vi "Configure Capture Analyzer Measurement Write To File.vi"(8 "error in (no error)":errorcluster, 9 "Write to File (Off)":bool, 10 "Instance (1)":i32=1, 11 "VISA resource name":refnum<visa-resource-name>) -> (0 "error out":errorcluster, 3 "VISA resource name out":refnum<visa-resource-name>)   [LabVIEW 2015, in "Rohde&Schwarz CMXP GPRF.lvlib"]
doc: "Enables or disables saving of all buffer contents to files (I/Q data for all segments).\nWith <WriteToFolder> = ON, the files are stored when the capture buffer analyzer is started.\n\nAttribute:\nRSCMXPGPRF_ATTR_CAPTURE_ANALYZER_MEASUREMENT_WRITE_TO_FILE\n\nRemote-control command:\nCONFigure:GPRF:MEAS<i>:CANalyzer:SALL:WTFolder"
uses:
  <instrlib>/Rohde&Schwarz CMXP GPRF/Rohde&Schwarz CMXP GPRF.lvlib
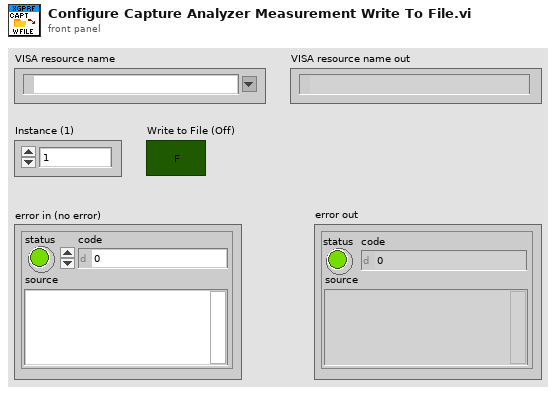
[diagram p1: front panel]
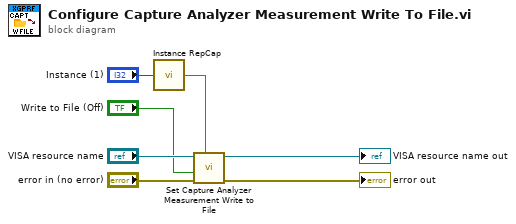
[diagram p0: block diagram]
diagram:
  n1 = call <instrlib>:"Instance RepCap.vi"("instance  in"="Instance (1)") -> ("instance out"=w2:string)
  n2 = call "Set Capture Analyzer Measurement Write to File"("Repeated Capabilities"=w2, "error in (no error)"="error in (no error)", "Capture Analyzer Measurement Write to File (OFF)"="Write to File (Off)", "instrument handle"="VISA resource name") -> ("error out"=→"error out":errorcluster, "instrument handle out"=→"VISA resource name out":refnum<visa-resource-name>)  [unwired: 6 in]
